vi "ColorScale.vi"(8 "error in (no error)":errorcluster, 11 "ITX Commands in":refnum<class "ITX Commands.lvclass">) -> (0 "error out":errorcluster, 3 "ITX Commands out":refnum<class "ITX Commands.lvclass">)   [LabVIEW 2016, in "ITX Commands.lvclass"]
uses:
  ITX Commands.lvclass
  ITX Commands.lvclass/ITX Commands.ctl
panel:
  out "resulting string":string="ModifyImage '' ctab{,, Rainbow, 0}"
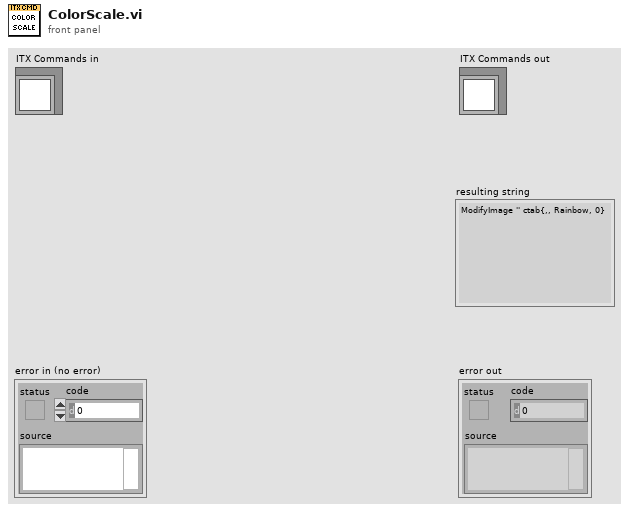
[diagram p1: front panel]
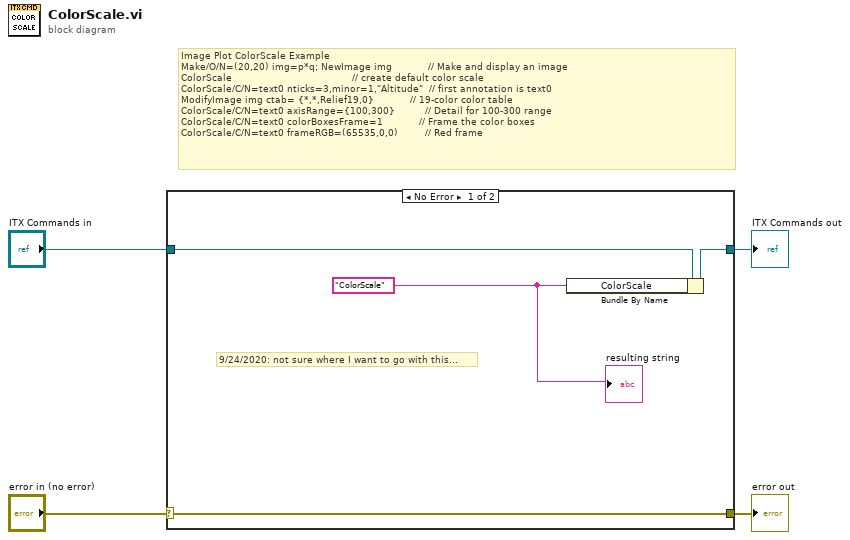
[diagram p0: block diagram]
diagram:
  # "Image Plot ColorScale Example\nMake/O/N=(20,20) img=p*q; NewImage img\t\t\t         // Make and display an image\nColorScale\t\t\t\t\t\t                                  // create default color scale\nColorScale/C/N=text0 nticks=3,minor=1,\"Altitude\"\t // first annotation is text0\nModifyImage img ctab= {*,*,Relief19,0}\t\t\t         // 19-color color table\nColorScale/C/N=text0 axisRange={100,300}\t\t        // Detail for 100-300 range\nColorScale/C/N=text0 colorBoxesFrame=1\t\t\t         // Frame the color boxes\nColorScale/C/N=text0 frameRGB=(65535,0,0)\t\t       // Red frame"
  n1 = case shown="No Error" "error in (no error)" {
    selector: "error in (no error)" -> [w5 w10]
    tunnel: [w5 w10] -> w3
    tunnel: [w7 w9] -> w1
    tunnel: "ITX Commands in" -> [w8 w9]
    frame No Error {
      w6 = "ColorScale" ("format string")
      # "9/24/2020: not sure where I want to go with this..."
      n2 = Bundle By Name(cluster=w8, "ColorScale"=w6) -> (w7:refnum<class "ITX Commands.lvclass">)
      "resulting string" <- w6
    }
    frame Error {
    }
  }
  "error out" <- w3
  "ITX Commands out" <- w1
